vi "TAT_Varient Creater.vi"(8 "error in (no error)":errorcluster) -> (0 "error out":errorcluster)   [LabVIEW 2017]
uses:
  <vilib>/Utility/miscctls.llb/LVRangeTypeDef.ctl
  <vilib>/addons/database/Connection.llb/Conn ObjectReference.ctl
  <vilib>/Utility/miscctls.llb/LVRowAndColumnUnsignedTypeDef.ctl
  b1939813-2d0c-4b6e-8ee7-2e1edd5edc28.vi
  <vilib>/Utility/config.llb/Read Key (I32).vi
  <vilib>/Utility/config.llb/Read Key (String).vi
  <vilib>/Utility/config.llb/Write Key (U32).vi
  <vilib>/Utility/config.llb/Write Key (String).vi
  <vilib>/Utility/config.llb/NI_LVConfig.lvlib
  <vilib>/addons/database/NI_Database_API.lvlib
panel:
  in  "BOX WEIGHT":u16=1 min=1 max=100 step=1 format="%.0f gm"
  in  "BOX RH PART QUANTITY":u16=1 min=1 max=100 step=1
  in  "BOX LH PART QUANTITY":u16=1 min=1 max=100 step=1
  in  "BOX CODE PREFIX":string
  in  "RH CODE PREFIX":string
  in  "Vertical Slider Control":dbl(slide)=1.0
  in  "CANCLE 3":bool
  in  "PRINTING":bool
  in  "Manual print":bool
  in  "Cancle 2":bool
  in  "Delete Button":bool
  in  "Cancle":bool
  in  "Save Button":bool
  in  "LH CODE PREFIX":string
  in  "Delete Square":bool
  in  "EDIT & SAVE":bool
  out "Varient Details":string[][](table)
  in  "PART NUMBER":u16=1 min=1 max=100 step=1
  in  "HOME":bool
  in  "UPDATE TABLE":bool
  in  "PART NAME":string(combo)
  # "Varient Creater"
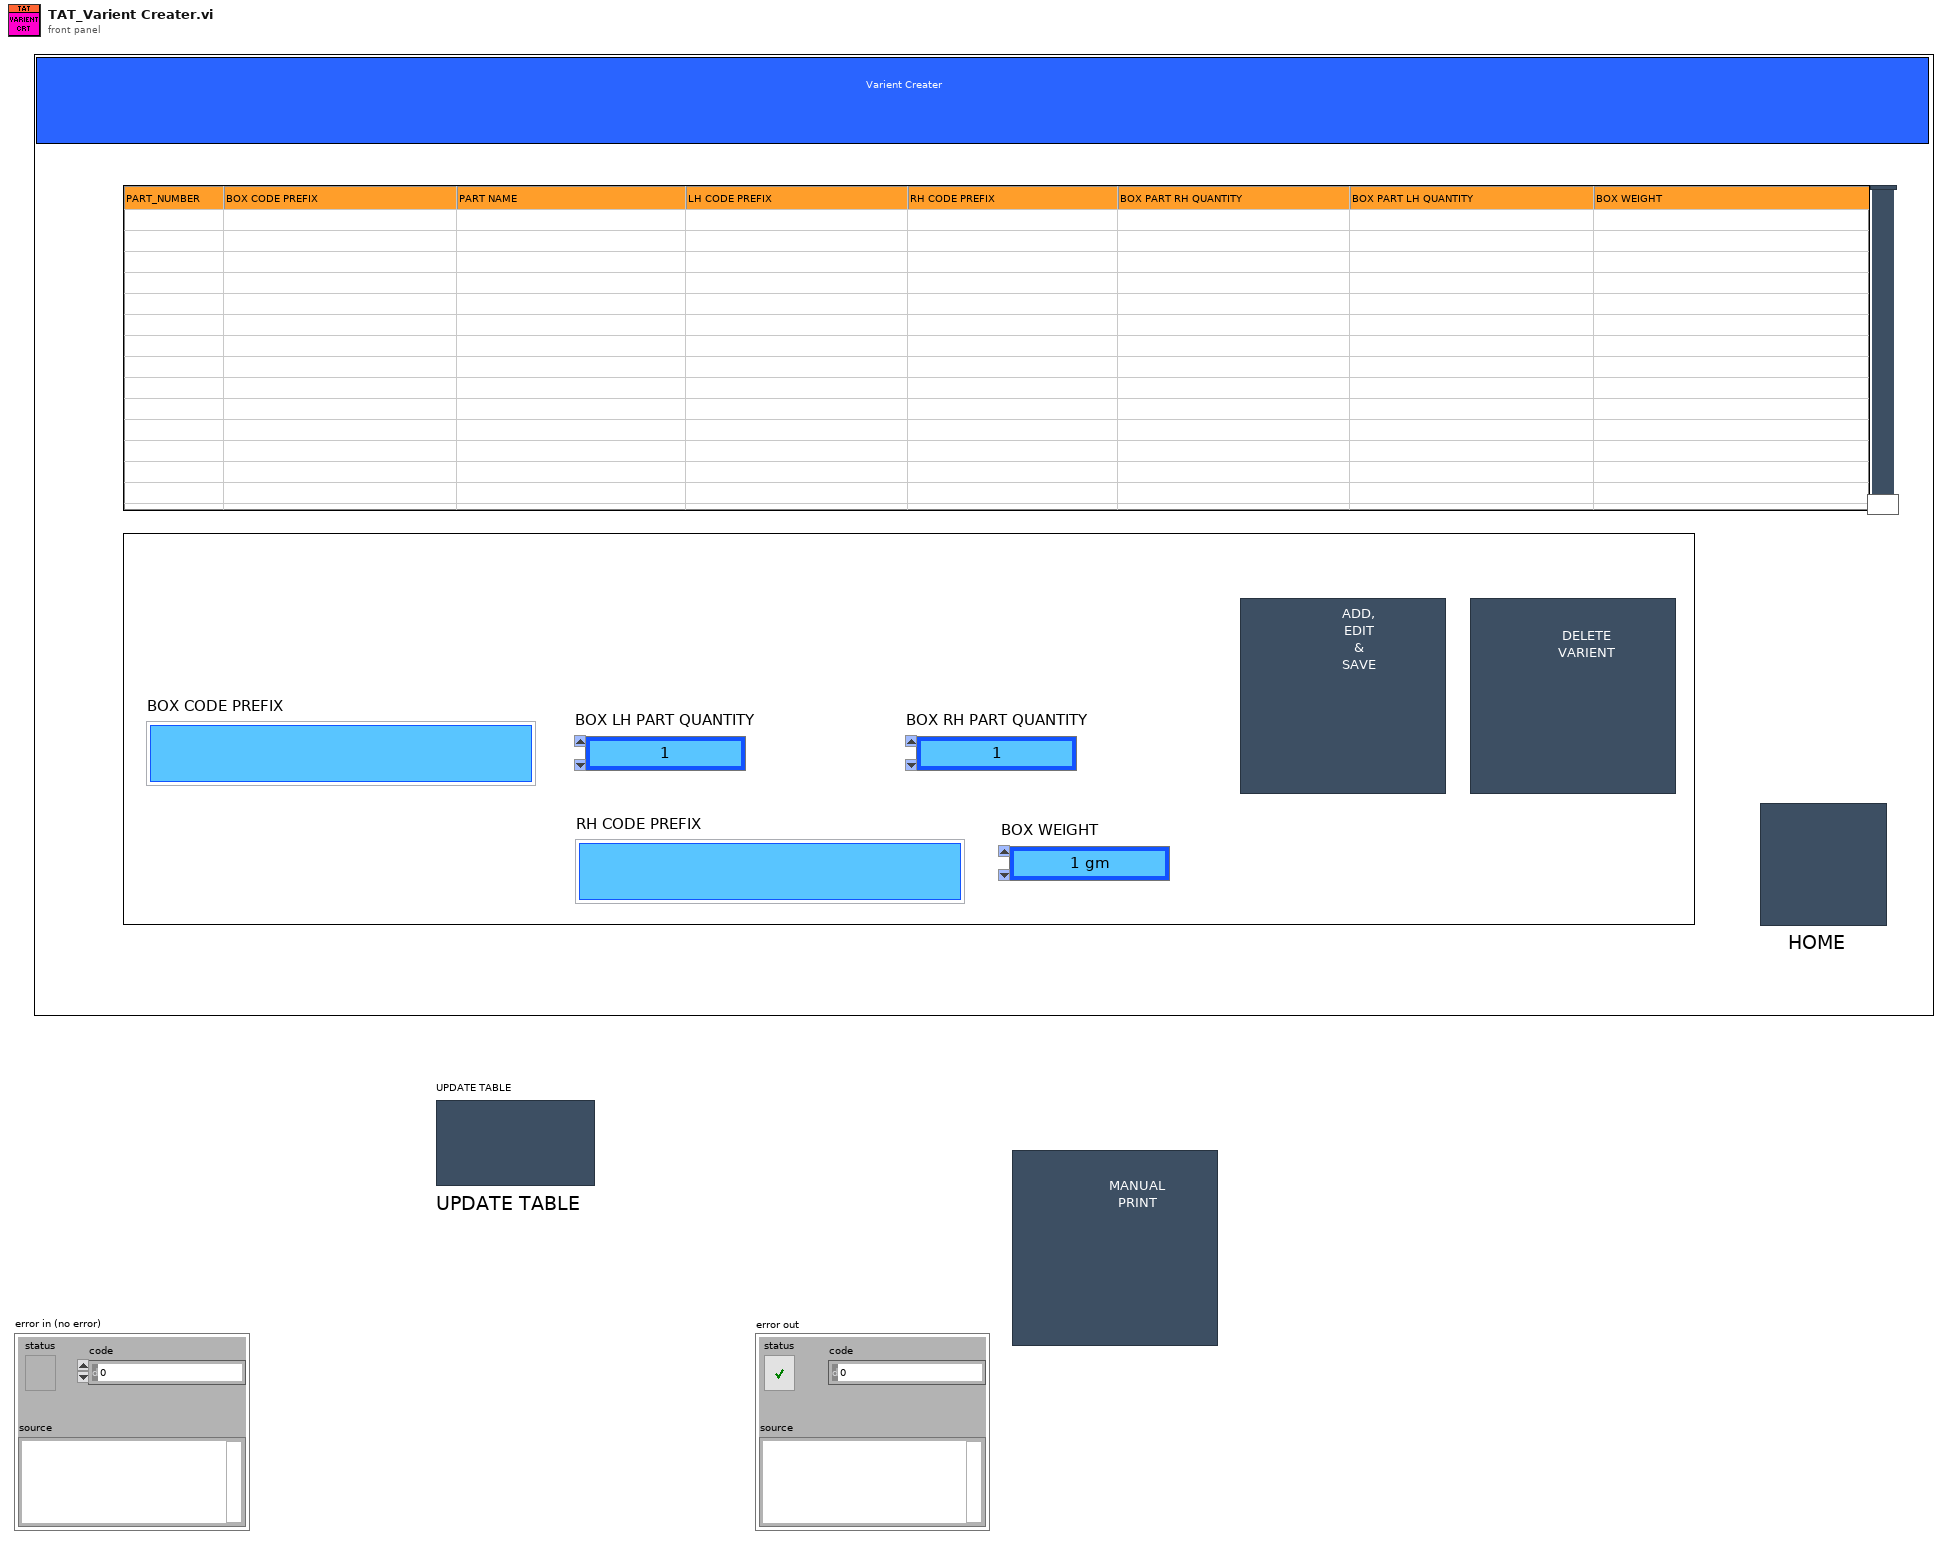
[diagram p1: front panel]
types:
  T1 = enum8{"Enabled", "Disabled", "Disabled and Grayed Out"}
  T2 = enum32{"invalid app kind", "Development System", "Run Time System", "Student Edition", "Embedded LabVIEW", "Evaluation", "Custom"}
  T3 = typedef "NI_LVConfig.lvlib/Config Data RefNum.ctl" = refnum<k1>
  T4 = typedef "LVRangeTypeDef.ctl" = cluster{"Minimum":dbl, "Maximum":dbl, "Increment":dbl, "Minor Increment":dbl, "Start":dbl}
  T5 = typedef "NI_Database_API.lvlib/Conn ObjectReference.ctl" = refnum<k1>
  T6 = cluster{"Varient number":u16, "Part name":string, "connection reference":T5, "Batch_Size":u16, "PART_NO":string, "TORISHI_CODE":string, "scanner com":refnum<visa-resource-name>, "Part Name List":string[], "Varient path":path, "Current Varient path":path, "Communication path":path, "Package path":path, "Part PRN path":path, "Station2 printer IP":string, "Station1 printer IP":string, "Current Serial Number":string, "Station1_QR":string, "Serial_Number":path, "PRIVIOUS code":string[], "Barcode station2 log":string, "Barcode station2 Up":string, "HARNESS CODE":string, "Station 1 bypass":bool}
  T7 = typedef "LVRowAndColumnUnsignedTypeDef.ctl" = cluster{"Row":u32, "Column":u32}
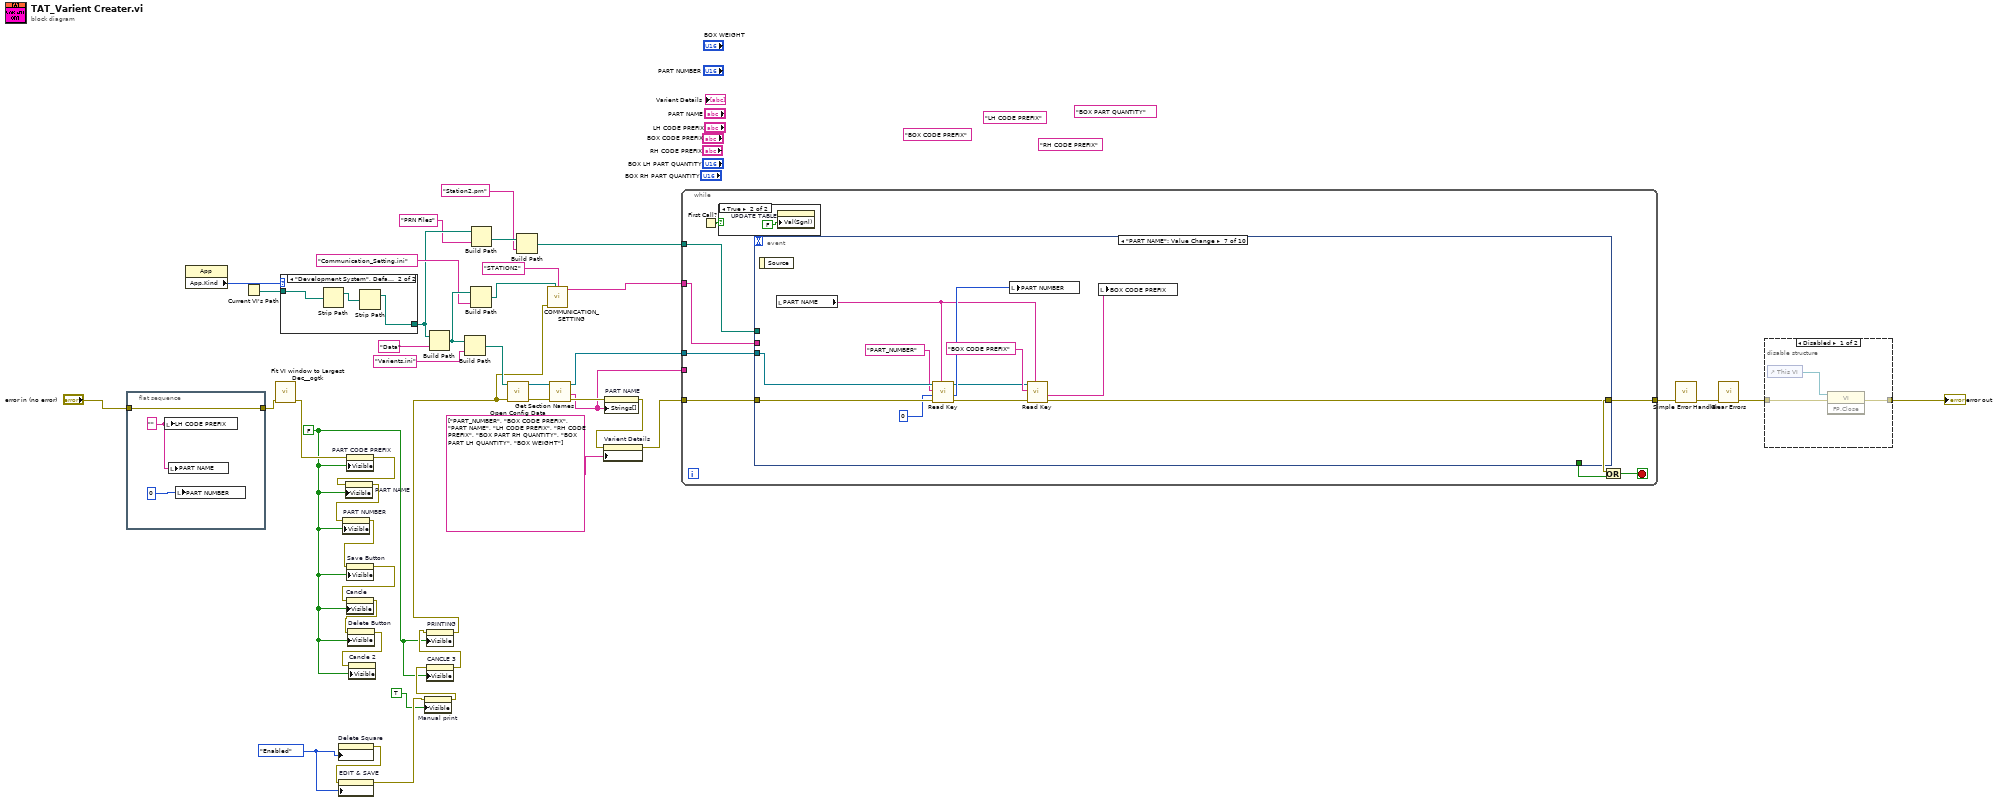
[diagram p0: block diagram]
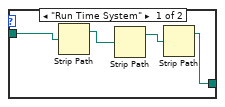
[diagram p3: hidden frame]
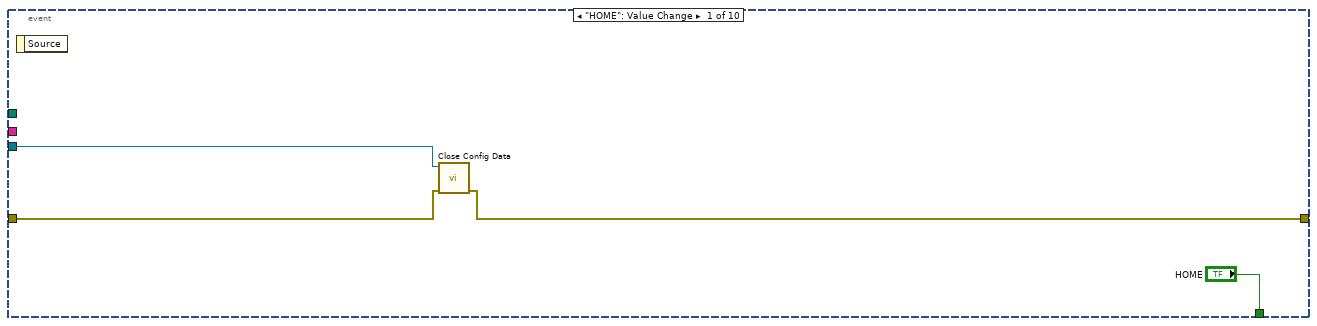
[diagram p5: hidden frame]
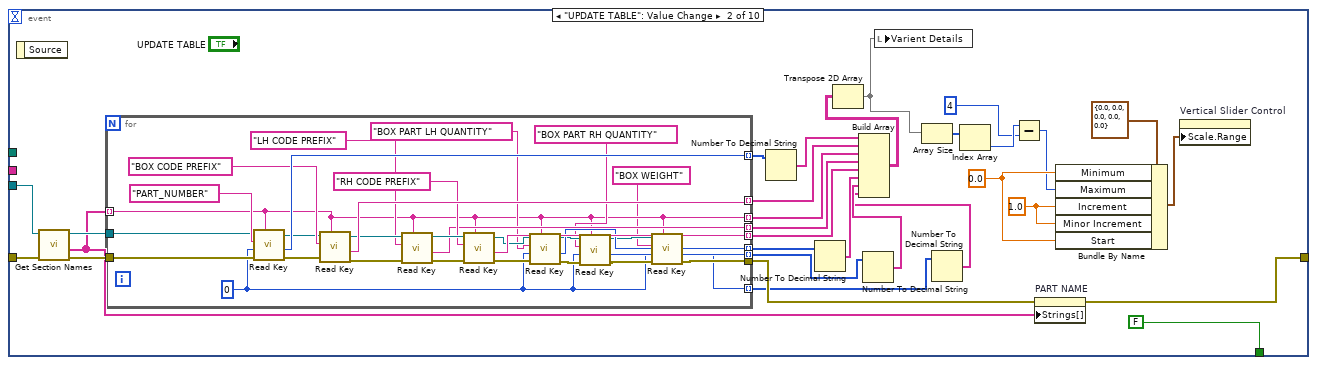
[diagram p6: hidden frame]
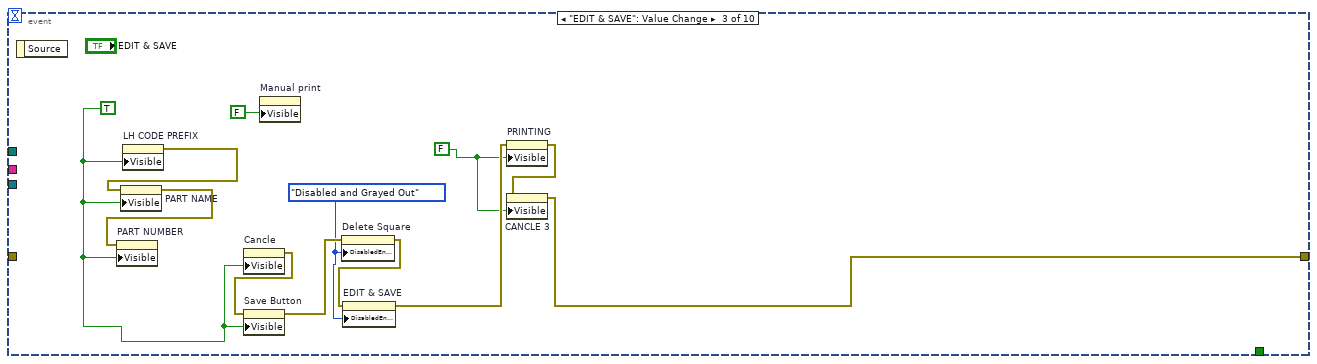
[diagram p7: hidden frame]
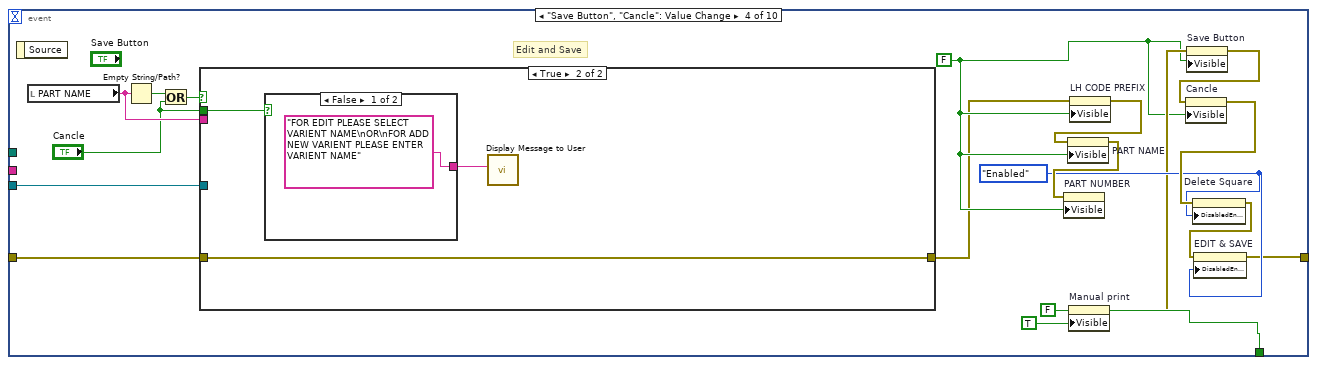
[diagram p8: hidden frame]
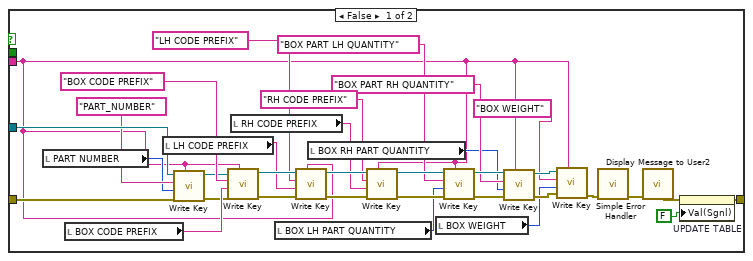
[diagram p9: hidden frame]
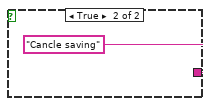
[diagram p10: hidden frame]
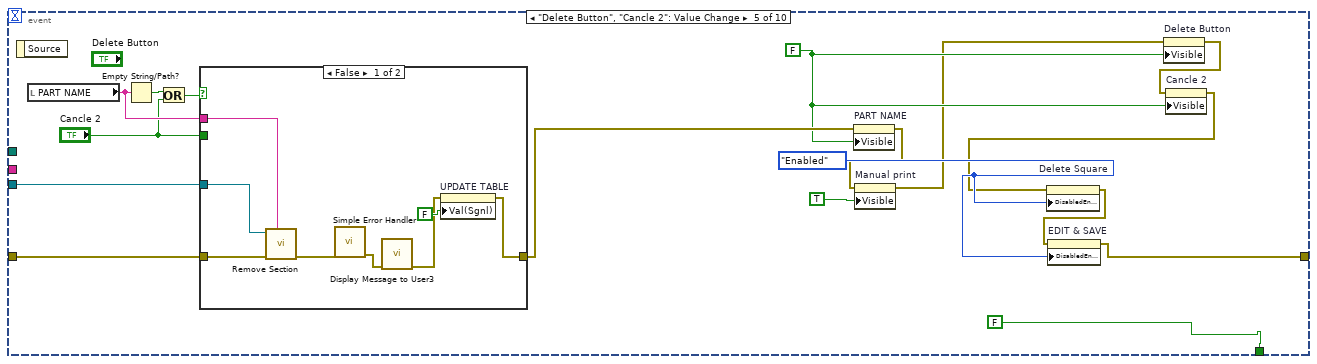
[diagram p11: hidden frame]
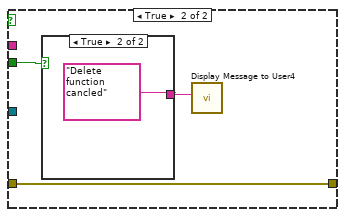
[diagram p12: hidden frame]
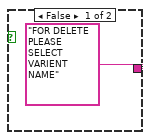
[diagram p13: hidden frame]
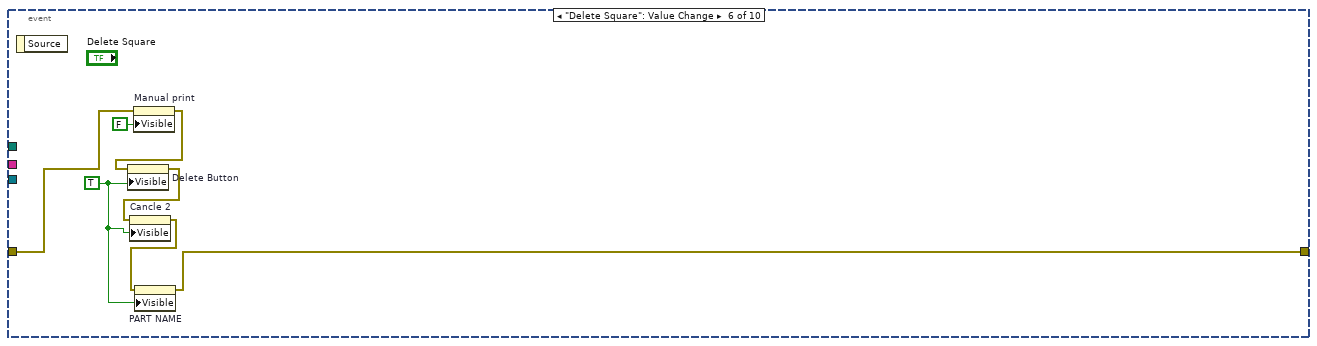
[diagram p14: hidden frame]
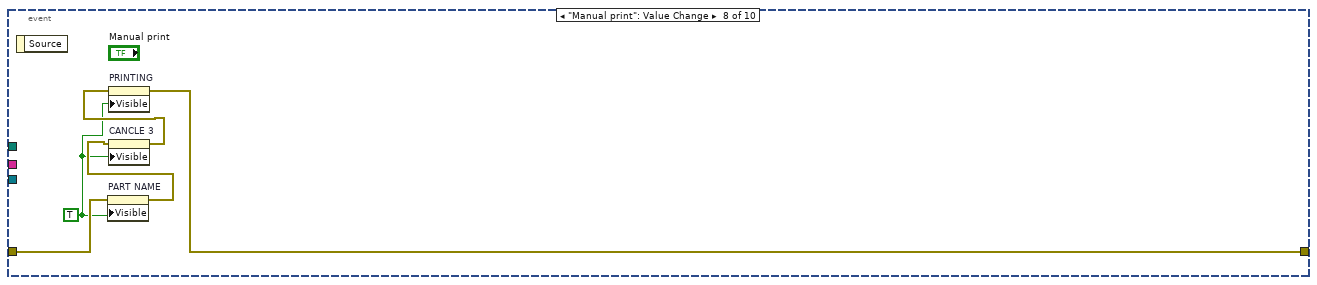
[diagram p15: hidden frame]
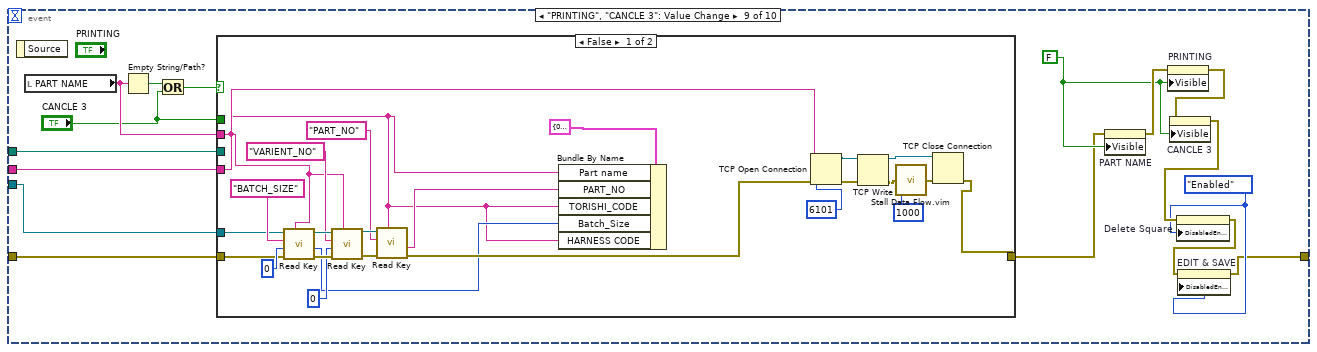
[diagram p16: hidden frame]
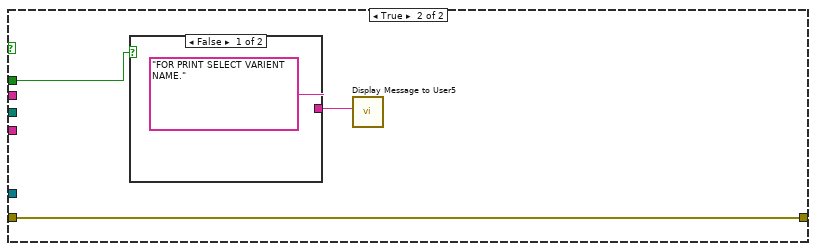
[diagram p17: hidden frame]
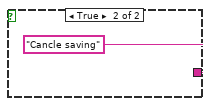
[diagram p18: hidden frame]
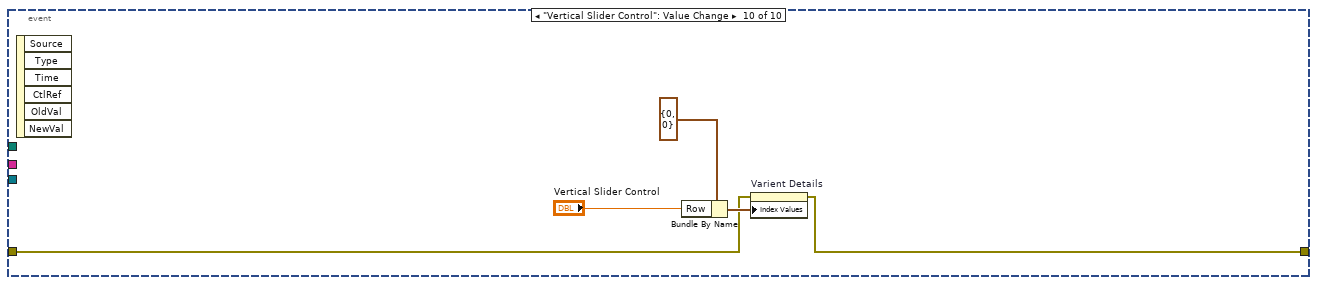
[diagram p19: hidden frame]
diagram:
  (unwired) "BOX PART QUANTITY" ("key")
  (unwired) "RH CODE PREFIX" ("key")
  (unwired) "LH CODE PREFIX" ("key")
  (unwired) "BOX CODE PREFIX" ("key")
  w20 = T1."Enabled" ("Disabled")
  w1 = FALSE
  n1 = flat-sequence {
    tunnel: [w45] -> w26
    tunnel: "error in (no error)" -> [w45]
    frame #0 {
      w47 = "" ("PART NUMBER")
      n2 = local write "LH CODE PREFIX"(w47) -> ()
      n3 = local write "PART NAME"(w47) -> ()
      n4 = local write "PART NUMBER"(u16 0 ("BATCH SIZE")) -> ()
    }
  }
  n5 = property class="App"() -> ("App.Kind"=w39:T2)  [unwired: 2 in, 2 out]
  n6 = Current VI's Path() -> (path=w40:path)
  n7 = call <userlib>:"Fit VI window to Largest Dec__ogtk.vi"("error in (no error)"=w26) -> ("error out"=w22:errorcluster)  [unwired: 5 in, 1 out]
  n8 = case shown="\"Development System\", Default" w39 {
    tunnel: w40 -> [w49 w53]
    tunnel: [w48 w52] -> w6
    frame "Run Time System" {
      n9 = Strip Path(path=w49) -> (stripped path=w51:path)  [unwired: 1 out]
      n10 = Strip Path(path=w51) -> (stripped path=w50:path)  [unwired: 1 out]
      n11 = Strip Path(path=w50) -> (stripped path=w48:path)  [unwired: 1 out]
    }
    frame "Development System", Default {
      n12 = Strip Path(path=w53) -> (stripped path=w54:path)  [unwired: 1 out]
      n13 = Strip Path(path=w54) -> (stripped path=w52:path)  [unwired: 1 out]
    }
  }
  n14 = property on="Delete Square" class="Bool"("DisabledEnum"=w20) -> (error out=w21:errorcluster)  [unwired: 2 in, 1 out]
  n15 = property on="EDIT & SAVE" class="Bool"(error in=w21, "DisabledEnum"=w20) -> (error out=w15:errorcluster)  [unwired: 1 in, 1 out]
  n16 = property on="PART CODE PREFIX" class="Str"(error in=w22, "Visible"=w1) -> (error out=w25:errorcluster)  [unwired: 1 in, 1 out]
  n17 = property on="PART NAME" class="CmbBox"(error in=w25, "Visible"=w1) -> (error out=w24:errorcluster)  [unwired: 1 in, 1 out]
  n18 = property on="PART NUMBER" class="DigNum (strict)"(error in=w24, "Visible"=w1) -> (error out=w23:errorcluster)  [unwired: 1 in, 1 out]
  n19 = property on="Save Button" class="Bool"(error in=w23, "Visible"=w1) -> (error out=w19:errorcluster)  [unwired: 1 in, 1 out]
  n20 = property on="Cancle" class="Bool"(error in=w19, "Visible"=w1) -> (error out=w18:errorcluster)  [unwired: 1 in, 1 out]
  n21 = property on="Delete Button" class="Bool"(error in=w18, "Visible"=w1) -> (error out=w17:errorcluster)  [unwired: 1 in, 1 out]
  n22 = property on="Cancle 2" class="Bool"(error in=w17, "Visible"=w1) -> ()  [unwired: 1 in, 2 out]
  n23 = property on="Manual print" class="Bool"(error in=w15, "Visible"=TRUE) -> (error out=w14:errorcluster)  [unwired: 1 in, 1 out]
  n24 = property on="CANCLE 3" class="Bool"(error in=w14, "Visible"=w1) -> (error out=w16:errorcluster)  [unwired: 1 in, 1 out]
  n25 = property on="PRINTING" class="Bool"(error in=w16, "Visible"=w1) -> (error out=w8:errorcluster)  [unwired: 1 in, 1 out]
  n26 = Build Path(base path=w6, name or relative path="Data") -> (appended path=w12:path)
  n27 = Build Path(base path=w12, name or relative path="Varients.ini") -> (appended path=w38:path)
  n28 = Build Path(base path=w12, name or relative path="Communication_Setting.ini") -> (appended path=w9:path)
  n29 = Build Path(base path=w6, name or relative path="PRN Files") -> (appended path=w4:path)
  n30 = call <vilib>:"Open Config Data.vi"("error in (no error)"=w8, "configuration file path"=w38) -> ("error out"=w34:errorcluster, "refnum"=w35:T3)  [unwired: 7 in, 1 out]
  n31 = Build Path(base path=w4, name or relative path="Station2.prn") -> (appended path=w2:path)
  n32 = call "COMMUNICATION_SETTING.vi"("communication path"=w9, "error in"=w8, "STATION"="STATION2") -> ("PRINT_COM"=w7:string)  [unwired: 6 in, 2 out]
  n33 = call <vilib>:"Get Section Names.vi"("error in (no error)"=w34, "refnum"=w35) -> ("error out"=w33:errorcluster, "section names"=w28:string[], "refnum out"=w32:T3)  [unwired: 7 in]
  n34 = property on="PART NAME" class="CmbBox"(error in=w33, "Strings[]"=w28) -> (error out=w31:errorcluster)  [unwired: 1 in, 1 out]
  n35 = property on="Varient Details" class="Tbl (strict)"(error in=w31, "Column Headers[]"=string[] ["PART_NUMBER", "BOX CODE PREFIX", "PART NAME", "LH CODE PREFIX", "RH CODE PREFIX", "BOX PART RH QUANTITY", "BOX PART LH QUANTITY", "BOX WEIGHT"] ("Column Header Strings[]")) -> (error out=w30:errorcluster)  [unwired: 1 in, 1 out]
  n36 = while {
    tunnel: w30 -> [w61]
    tunnel: [w59] -> w41
    tunnel: w32 -> [w58]
    tunnel: w28 -> [_]
    tunnel: w7 -> [w56]
    tunnel: w2 -> [w55]
    stop <- w60 stop-if-true
    n37 = First Call?() -> (First Call?: T/F=w57:bool)
    n38 = case shown="True" w57 {
      frame False {
      }
      frame True {
        n39 = property on="UPDATE TABLE" class="Bool (strict)"("Val(Sgnl)"=FALSE) -> ()  [unwired: 2 in, 2 out]
      }
    }
    n40 = event shown="[6] \"PART NAME\": Value Change" {
      selector: _ -> [_ _ _ _ _ _ _ _ _ _]
      dyn-events: _ -> [_ _ _ _ _ _ _ _ _ _]
      timeout: _ -> [_ _ _ _ _ _ _ _ _ _]
      tunnel: ["HOME" FALSE ("stop") _ FALSE ("stop") FALSE ("stop") _ _ _ _ _] -> w62
      tunnel: w61 -> [w66 w94 _ w156 w212 w229 w245 w248 w266 w297]
      tunnel: [w65 w88 w131 w145 w204 w232 w237 w247 w255 w298] -> w59
      tunnel: w58 -> [w64 w92 _ w157 w213 _ w244 _ w262 _]
      tunnel: w56 -> [_ _ _ _ _ _ _ _ w253 _]
      tunnel: w55 -> [_ _ _ _ _ _ _ _ w252 _]
      event "HOME": Value Change {
        n41 = event-data() -> ()  [unwired: 1 in, 1 out]
        n42 = call <vilib>:"Close Config Data.vi"("error in (no error)"=w66, "refnum"=w64) -> ("error out"=w65:errorcluster)  [unwired: 8 in, 1 out]
      }
      event "UPDATE TABLE": Value Change {
        w85 = 1.0 ("Increment")
        w84 = 0.0 ("Minimum")
        n43 = event-data() -> ()  [unwired: 1 in, 1 out]
        n44 = call <vilib>:"Get Section Names.vi"("error in (no error)"=w94, "refnum"=w92) -> ("error out"=w93:errorcluster, "section names"=w89:string[], "refnum out"=w91:T3)  [unwired: 7 in]
        n45 = for {
          tunnel: [w103] -> w90
          tunnel: w93 -> [w127]
          tunnel: w89 -> [w101] mode=indexing
          tunnel: w91 -> [w126]
          tunnel: [w125] -> w96 mode=indexing
          tunnel: [w121] -> w77 mode=indexing
          tunnel: [w101] -> w76 mode=indexing
          tunnel: [w114] -> w75 mode=indexing
          tunnel: [w113] -> w74 mode=indexing
          tunnel: [w108] -> w72 mode=indexing
          tunnel: [w106] -> w70 mode=indexing
          tunnel: [w98] -> w68 mode=indexing
          w99 = 0 ("default value")
          n46 = call-poly <vilib>:"Read Key.vi"("section"=w101, "error in (no error)"=w127, "default value"=w99, "key"="PART_NUMBER", "refnum"=w126) -> ("error out"=w124:errorcluster, "value"=w125:i32, "refnum out"=w122:T3)  [unwired: 3 in, 1 out]
          n47 = call-poly <vilib>:"Read Key.vi"("section"=w101, "error in (no error)"=w124, "key"="BOX CODE PREFIX", "refnum"=w122) -> ("error out"=w116:errorcluster, "value"=w121:string, "refnum out"=w120:T3)  [unwired: 4 in, 1 out]
          n48 = call-poly <vilib>:"Read Key.vi"("section"=w101, "error in (no error)"=w116, "key"="LH CODE PREFIX", "refnum"=w120) -> ("error out"=w117:errorcluster, "value"=w114:string, "refnum out"=w118:T3)  [unwired: 4 in, 1 out]
          n49 = call-poly <vilib>:"Read Key.vi"("section"=w101, "error in (no error)"=w117, "key"="RH CODE PREFIX", "refnum"=w118) -> ("error out"=w112:errorcluster, "value"=w113:string, "refnum out"=w111:T3)  [unwired: 4 in, 1 out]
          n50 = call-poly <vilib>:"Read Key.vi"("section"=w101, "error in (no error)"=w112, "default value"=w99, "key"="BOX PART LH QUANTITY", "refnum"=w111) -> ("error out"=w109:errorcluster, "value"=w108:i32, "refnum out"=w107:T3)  [unwired: 3 in, 1 out]
          n51 = call-poly <vilib>:"Read Key.vi"("section"=w101, "error in (no error)"=w109, "default value"=w99, "key"="BOX PART RH QUANTITY", "refnum"=w107) -> ("error out"=w104:errorcluster, "value"=w106:i32, "refnum out"=w102:T3)  [unwired: 3 in, 1 out]
          n52 = call-poly <vilib>:"Read Key.vi"("section"=w101, "error in (no error)"=w104, "default value"=w99, "key"="BOX WEIGHT", "refnum"=w102) -> ("error out"=w103:errorcluster, "value"=w98:i32)  [unwired: 3 in, 2 out]
        }
        n53 = Number To Decimal String(number=w96) -> (decimal integer string=w78:string[])  [unwired: 1 in]
        n54 = Number To Decimal String(number=w72) -> (decimal integer string=w73:string[])  [unwired: 1 in]
        n55 = Number To Decimal String(number=w70) -> (decimal integer string=w71:string[])  [unwired: 1 in]
        n56 = Number To Decimal String(number=w68) -> (decimal integer string=w69:string[])  [unwired: 1 in]
        n57 = Build Array(w78, w77, w76, w75, w74, w73, w71, w69) -> (w95:string[][])
        n58 = Transpose 2D Array(2D array=w95) -> (transposed array=w87:string[][])
        n59 = local write "Varient Details"(w87) -> ()
        n60 = Array Size(array=w87) -> (size(s)=w86:i32[])
        n61 = Index Array(array=w86) -> (element=w81:i32)  [unwired: 1 in]
        n62 = Subtract(x=w81, y=4) -> (x-y=w80:i32)
        n63 = property on="PART NAME" class="CmbBox"(error in=w90, "Strings[]"=w89) -> (error out=w88:errorcluster)  [unwired: 1 in, 1 out]
        n64 = Bundle By Name(cluster=T4 {"Minimum"=0.0, "Maximum"=0.0, "Increment"=0.0, "Minor Increment"=0.0, "Start"=0.0} ("Scale.Range"), "Minimum"=w84, "Maximum"=w80, "Increment"=w85, "Minor Increment"=w85, "Start"=w84) -> (w83:T4)
        n65 = property on="Vertical Slider Control" class="Slide (strict)"("Scale.Range"=w83) -> ()  [unwired: 2 in, 2 out]
      }
      event "EDIT & SAVE": Value Change {
        w130 = FALSE
        w136 = T1."Disabled and Grayed Out" ("Disabled")
        w129 = TRUE
        n66 = event-data() -> ()  [unwired: 1 in, 1 out]
        n67 = property on="LH CODE PREFIX" class="Str"("Visible"=w129) -> (error out=w139:errorcluster)  [unwired: 2 in, 1 out]
        n68 = property on="PART NAME" class="CmbBox"(error in=w139, "Visible"=w129) -> (error out=w140:errorcluster)  [unwired: 1 in, 1 out]
        n69 = property on="PART NUMBER" class="DigNum (strict)"(error in=w140, "Visible"=w129) -> ()  [unwired: 1 in, 2 out]
        n70 = property on="Cancle" class="Bool"("Visible"=w129) -> (error out=w135:errorcluster)  [unwired: 2 in, 1 out]
        n71 = property on="Save Button" class="Bool"(error in=w135, "Visible"=w129) -> (error out=w138:errorcluster)  [unwired: 1 in, 1 out]
        n72 = property on="Manual print" class="Bool"("Visible"=FALSE) -> ()  [unwired: 2 in, 2 out]
        n73 = property on="Delete Square" class="Bool"(error in=w138, "DisabledEnum"=w136) -> (error out=w137:errorcluster)  [unwired: 1 in, 1 out]
        n74 = property on="EDIT & SAVE" class="Bool"(error in=w137, "DisabledEnum"=w136) -> (error out=w132:errorcluster)  [unwired: 1 in, 1 out]
        n75 = property on="PRINTING" class="Bool"(error in=w132, "Visible"=w130) -> (error out=w133:errorcluster)  [unwired: 1 in, 1 out]
        n76 = property on="CANCLE 3" class="Bool"(error in=w133, "Visible"=w130) -> (error out=w131:errorcluster)  [unwired: 1 in, 1 out]
      }
      event "Save Button", "Cancle": Value Change {
        w146 = T1."Enabled" ("Disabled")
        w142 = FALSE
        # "Edit and Save"
        n77 = event-data() -> ()  [unwired: 1 in, 1 out]
        n78 = local read "PART NAME"() -> (w155:string)
        n79 = Empty String/Path?(string/path=w155) -> (empty?=w154:bool)
        n80 = Or(x=w154, y="Cancle") -> (x .or. y?=w153:bool)
        n81 = case shown="True" w153 {
          tunnel: w156 -> [w192 w195]
          tunnel: [w188 w195] -> w141
          tunnel: w157 -> [w191 _]
          tunnel: w155 -> [w161 _]
          tunnel: "Cancle" -> [_ w193]
          frame False {
            n82 = local read "PART NUMBER"() -> (w187:u16)
            n83 = local read "BOX CODE PREFIX"() -> (w183:string)
            n84 = local read "LH CODE PREFIX"() -> (w169:string)
            n85 = call-poly <vilib>:"Write Key.vi"("section"=w161, "error in (no error)"=w192, "value"=w187, "key"="PART_NUMBER", "refnum"=w191) -> ("error out"=w181:errorcluster, "refnum out"=w182:T3)  [unwired: 4 in, 1 out]
            n86 = call-poly <vilib>:"Write Key.vi"("section"=w161, "error in (no error)"=w181, "value"=w183, "key"="BOX CODE PREFIX", "refnum"=w182) -> ("error out"=w180:errorcluster, "refnum out"=w179:T3)  [unwired: 4 in, 1 out]
            n87 = local read "RH CODE PREFIX"() -> (w170:string)
            n88 = local read "BOX LH PART QUANTITY"() -> (w171:u16)
            n89 = call-poly <vilib>:"Write Key.vi"("section"=w161, "error in (no error)"=w180, "value"=w169, "key"="LH CODE PREFIX", "refnum"=w179) -> ("error out"=w178:errorcluster, "refnum out"=w177:T3)  [unwired: 4 in, 1 out]
            n90 = local read "BOX RH PART QUANTITY"() -> (w165:u16)
            n91 = call-poly <vilib>:"Write Key.vi"("section"=w161, "error in (no error)"=w178, "value"=w170, "key"="RH CODE PREFIX", "refnum"=w177) -> ("error out"=w176:errorcluster, "refnum out"=w175:T3)  [unwired: 4 in, 1 out]
            n92 = local read "BOX WEIGHT"() -> (w159:u16)
            n93 = call-poly <vilib>:"Write Key.vi"("section"=w161, "error in (no error)"=w176, "value"=w171, "key"="BOX PART LH QUANTITY", "refnum"=w175) -> ("error out"=w167:errorcluster, "refnum out"=w168:T3)  [unwired: 4 in, 1 out]
            n94 = call-poly <vilib>:"Write Key.vi"("section"=w161, "error in (no error)"=w167, "value"=w165, "key"="BOX PART RH QUANTITY", "refnum"=w168) -> ("error out"=w163:errorcluster, "refnum out"=w164:T3)  [unwired: 4 in, 1 out]
            n95 = call-poly <vilib>:"Write Key.vi"("section"=w161, "error in (no error)"=w163, "value"=w159, "key"="BOX WEIGHT", "refnum"=w164) -> ("error out"=w162:errorcluster)  [unwired: 4 in, 2 out]
            n96 = call <vilib>:"Simple Error Handler.vi"("error in (no error)"=w162) -> ("error out"=w186:errorcluster)  [unwired: 4 in, 4 out]
            n97 = call "Display Message to User2"("error in (no error)"=w186) -> ("error out"=w185:errorcluster)  [unwired: 9 in, 1 out]
            n98 = property on="UPDATE TABLE" class="Bool (strict)"(error in=w185, "Val(Sgnl)"=FALSE) -> (error out=w188:errorcluster)  [unwired: 1 in, 1 out]
          }
          frame True {
            n99 = case shown="False" w193 {
              tunnel: ["FOR EDIT PLEASE SELECT VARIENT NAME\nOR\nFOR ADD NEW VARIENT PLEASE ENTER VARIENT NAME" "Cancle saving"] -> w194
              frame False {
              }
              frame True {
              }
            }
            n100 = call "Display Message to User"("Message"=w194) -> ()  [unwired: 9 in, 2 out]
          }
        }
        n101 = property on="Manual print" class="Bool"("Visible"=TRUE) -> (error out=w143:errorcluster)  [unwired: 2 in, 1 out]
        n102 = property on="LH CODE PREFIX" class="Str"(error in=w141, "Visible"=w142) -> (error out=w151:errorcluster)  [unwired: 1 in, 1 out]
        n103 = property on="PART NAME" class="CmbBox"(error in=w151, "Visible"=w142) -> (error out=w150:errorcluster)  [unwired: 1 in, 1 out]
        n104 = property on="PART NUMBER" class="DigNum (strict)"(error in=w150, "Visible"=w142) -> ()  [unwired: 1 in, 2 out]
        n105 = property on="Save Button" class="Bool"(error in=w143, "Visible"=w142) -> (error out=w148:errorcluster)  [unwired: 1 in, 1 out]
        n106 = property on="Cancle" class="Bool"(error in=w148, "Visible"=w142) -> (error out=w147:errorcluster)  [unwired: 1 in, 1 out]
        n107 = property on="Delete Square" class="Bool"(error in=w147, "DisabledEnum"=w146) -> (error out=w149:errorcluster)  [unwired: 1 in, 1 out]
        n108 = property on="EDIT & SAVE" class="Bool"(error in=w149, "DisabledEnum"=w146) -> (error out=w145:errorcluster)  [unwired: 1 in, 1 out]
      }
      event "Delete Button", "Cancle 2": Value Change {
        w206 = T1."Enabled" ("Disabled")
        w201 = FALSE
        n109 = event-data() -> ()  [unwired: 1 in, 1 out]
        n110 = local read "PART NAME"() -> (w211:string)
        n111 = Empty String/Path?(string/path=w211) -> (empty?=w210:bool)
        n112 = Or(x=w210, y="Cancle 2") -> (x .or. y?=w209:bool)
        n113 = case shown="False" w209 {
          tunnel: w212 -> [w216 w225]
          tunnel: [w221 w225] -> w205
          tunnel: w213 -> [w217 _]
          tunnel: w211 -> [w218 _]
          tunnel: "Cancle 2" -> [_ w224]
          frame False {
            n114 = call <vilib>:"Remove Section.vi"("section"=w218, "error in (no error)"=w216, "refnum"=w217) -> ("error out"=w215:errorcluster)  [unwired: 6 in, 2 out]
            n115 = call <vilib>:"Simple Error Handler.vi"("error in (no error)"=w215) -> ("error out"=w220:errorcluster)  [unwired: 4 in, 4 out]
            n116 = call "Display Message to User3"("error in (no error)"=w220) -> ("error out"=w219:errorcluster)  [unwired: 9 in, 1 out]
            n117 = property on="UPDATE TABLE" class="Bool (strict)"(error in=w219, "Val(Sgnl)"=FALSE) -> (error out=w221:errorcluster)  [unwired: 1 in, 1 out]
          }
          frame True {
            n118 = case shown="True" w224 {
              tunnel: ["FOR DELETE PLEASE SELECT VARIENT NAME" "Delete function cancled"] -> w223
              frame False {
              }
              frame True {
              }
            }
            n119 = call "Display Message to User4"("Message"=w223) -> ()  [unwired: 9 in, 2 out]
          }
        }
        n120 = property on="PART NAME" class="CmbBox"(error in=w205, "Visible"=w201) -> (error out=w199:errorcluster)  [unwired: 1 in, 1 out]
        n121 = property on="Manual print" class="Bool"(error in=w199, "Visible"=TRUE) -> (error out=w198:errorcluster)  [unwired: 1 in, 1 out]
        n122 = property on="Delete Button" class="Bool"(error in=w198, "Visible"=w201) -> (error out=w203:errorcluster)  [unwired: 1 in, 1 out]
        n123 = property on="Cancle 2" class="Bool"(error in=w203, "Visible"=w201) -> (error out=w202:errorcluster)  [unwired: 1 in, 1 out]
        n124 = property on="Delete Square" class="Bool"(error in=w202, "DisabledEnum"=w206) -> (error out=w207:errorcluster)  [unwired: 1 in, 1 out]
        n125 = property on="EDIT & SAVE" class="Bool"(error in=w207, "DisabledEnum"=w206) -> (error out=w204:errorcluster)  [unwired: 1 in, 1 out]
      }
      event "Delete Square": Value Change {
        w231 = TRUE
        n126 = event-data() -> ()  [unwired: 1 in, 1 out]
        n127 = property on="Manual print" class="Bool"(error in=w229, "Visible"=FALSE) -> (error out=w228:errorcluster)  [unwired: 1 in, 1 out]
        n128 = property on="Delete Button" class="Bool"(error in=w228, "Visible"=w231) -> (error out=w234:errorcluster)  [unwired: 1 in, 1 out]
        n129 = property on="Cancle 2" class="Bool"(error in=w234, "Visible"=w231) -> (error out=w233:errorcluster)  [unwired: 1 in, 1 out]
        n130 = property on="PART NAME" class="CmbBox"(error in=w233, "Visible"=w231) -> (error out=w232:errorcluster)  [unwired: 1 in, 1 out]
      }
      event "PART NAME": Value Change {
        n131 = event-data() -> ()  [unwired: 1 in, 1 out]
        n132 = local read "PART NAME"() -> (w236:string)
        n133 = call-poly <vilib>:"Read Key.vi"("section"=w236, "error in (no error)"=w245, "default value"=0, "key"="PART_NUMBER", "refnum"=w244) -> ("error out"=w240:errorcluster, "value"=w242:i32, "refnum out"=w238:T3)  [unwired: 3 in, 1 out]
        n134 = local write "PART NUMBER"(w242) -> ()
        n135 = call-poly <vilib>:"Read Key.vi"("section"=w236, "error in (no error)"=w240, "key"="BOX CODE PREFIX", "refnum"=w238) -> ("error out"=w237:errorcluster, "value"=w235:string)  [unwired: 4 in, 2 out]
        n136 = local write "BOX CODE PREFIX"(w235) -> ()
      }
      event "Manual print": Value Change {
        w246 = TRUE
        n137 = event-data() -> ()  [unwired: 1 in, 1 out]
        n138 = property on="PART NAME" class="CmbBox"(error in=w248, "Visible"=w246) -> (error out=w250:errorcluster)  [unwired: 1 in, 1 out]
        n139 = property on="CANCLE 3" class="Bool"(error in=w250, "Visible"=w246) -> (error out=w249:errorcluster)  [unwired: 1 in, 1 out]
        n140 = property on="PRINTING" class="Bool"(error in=w249, "Visible"=w246) -> (error out=w247:errorcluster)  [unwired: 1 in, 1 out]
      }
      event "PRINTING", "CANCLE 3": Value Change {
        w256 = T1."Enabled" ("Disabled")
        w257 = FALSE
        n141 = event-data() -> ()  [unwired: 1 in, 1 out]
        n142 = local read "PART NAME"() -> (w263:string)
        n143 = Empty String/Path?(string/path=w263) -> (empty?=w265:bool)
        n144 = Or(x=w265, y="CANCLE 3") -> (x .or. y?=w264:bool)
        n145 = case shown="False" w264 {
          tunnel: w266 -> [w282 w294]
          tunnel: [w273 w294] -> w254
          tunnel: w263 -> [w268 _]
          tunnel: w262 -> [w281 _]
          tunnel: w253 -> [w269 _]
          tunnel: w252 -> [_ _]
          tunnel: "CANCLE 3" -> [_ w292]
          frame False {
            n146 = call-poly <vilib>:"Read Key.vi"("section"=w268, "error in (no error)"=w282, "default value"=0, "key"="BATCH_SIZE", "refnum"=w281) -> ("error out"=w291:errorcluster, "value"=w272:i32, "refnum out"=w290:T3)  [unwired: 3 in, 1 out]
            n147 = call-poly <vilib>:"Read Key.vi"("section"=w268, "error in (no error)"=w291, "default value"=0, "key"="VARIENT_NO", "refnum"=w290) -> ("error out"=w288:errorcluster, "refnum out"=w287:T3)  [unwired: 3 in, 2 out]
            n148 = call-poly <vilib>:"Read Key.vi"("section"=w268, "error in (no error)"=w288, "key"="PART_NO", "refnum"=w287) -> ("error out"=w289:errorcluster, "value"=w270:string)  [unwired: 4 in, 2 out]
            n149 = Bundle By Name(cluster=T6 {"Varient number"=0, "Part name"="", "connection reference"=refnum, "Batch_Size"=0, "PART_NO"="", "TORISHI_CODE"="", "scanner com"="", "Part Name List"=[], "Varient path"=path "", "Current Varient path"=path "", "Communication path"=path "", "Package path"=path "", "Part PRN path"=path "", "Station2 printer IP"="", "Station1 printer IP"="", "Current Serial Number"="", "Station1_QR"="", "Serial_Number"=path "", "PRIVIOUS code"=[], "Barcode station2 log"="", "Barcode station2 Up"="", "HARNESS CODE"="", "Station 1 bypass"=FALSE} ("Cluster 2"), "Part name"=w268, "PART_NO"=w270, "TORISHI_CODE"=w268, "Batch_Size"=w272, "HARNESS CODE"=w268) -> ()  [unwired: 1 out]
            n150 = TCP Open Connection(address=w269, remote port or service name=u16 6101, error in (no error)=w289) -> (connection ID=w278:refnum<k5>, error out=w277:errorcluster)  [unwired: 2 in]
            n151 = TCP Write(connection ID=w278, error in (no error)=w277) -> (connection ID out=w280:refnum<k5>, error out=w276:errorcluster)  [unwired: 2 in, 1 out]
            n152 = call "Stall Data Flow.vim"("value in"=w276, "milliseconds to wait"=u32 1000) -> ("value out"=w279:errorcluster)  [unwired: 1 out]
            n153 = TCP Close Connection(connection ID=w280, error in (no error)=w279) -> (error out=w273:errorcluster)  [unwired: 1 in, 1 out]
          }
          frame True {
            n154 = case shown="False" w292 {
              tunnel: ["FOR PRINT SELECT VARIENT NAME." "Cancle saving"] -> w293
              frame False {
              }
              frame True {
              }
            }
            n155 = call "Display Message to User5"("Message"=w293) -> ()  [unwired: 9 in, 2 out]
          }
        }
        n156 = property on="PART NAME" class="CmbBox"(error in=w254, "Visible"=w257) -> (error out=w261:errorcluster)  [unwired: 1 in, 1 out]
        n157 = property on="PRINTING" class="Bool"(error in=w261, "Visible"=w257) -> (error out=w259:errorcluster)  [unwired: 1 in, 1 out]
        n158 = property on="CANCLE 3" class="Bool"(error in=w259, "Visible"=w257) -> (error out=w258:errorcluster)  [unwired: 1 in, 1 out]
        n159 = property on="Delete Square" class="Bool"(error in=w258, "DisabledEnum"=w256) -> (error out=w260:errorcluster)  [unwired: 1 in, 1 out]
        n160 = property on="EDIT & SAVE" class="Bool"(error in=w260, "DisabledEnum"=w256) -> (error out=w255:errorcluster)  [unwired: 1 in, 1 out]
      }
      event "Vertical Slider Control": Value Change {
        n161 = event-data() -> ()  [unwired: 1 in, 6 out]
        n162 = Bundle By Name(cluster=T7 {"Row"=0, "Column"=0} ("Index Values"), "Row"="Vertical Slider Control") -> (w300:T7)
        n163 = property on="Varient Details" class="Tbl (strict)"(error in=w297, "Index Values"=w300) -> (error out=w298:errorcluster)  [unwired: 1 in, 1 out]
      }
    }
    n164 = Or(x=w59, y=w62) -> (x .or. y?=w60:bool)
  }
  n165 = call <vilib>:"Simple Error Handler.vi"("error in (no error)"=w41) -> ("error out"=w44:errorcluster)  [unwired: 4 in, 4 out]
  n166 = call <vilib>:"Clear Errors.vi"("error in (no error)"=w44) -> ("error out"=w43:errorcluster)  [unwired: 5 in, 1 out]
  n167 = disable-structure shown="Disabled" {
    disable-tunnel: w43 -> [w304 w305]
    disable-tunnel: [w303 w305] -> w42
    frame Disabled {
      n168 = control-ref of="This VI"() -> (w302:refnum<vi>)
      n169 = invoke class="VI" method="FP.Close"(reference=w302, error in=w304) -> (error out=w303:errorcluster)  [unwired: 1 in, 2 out]
    }
    frame Enabled {
    }
  }
  "error out" <- w42
